vi "ge_RemoveArrayDup(String).vi"(4 "Input Array":string[](array[string])) -> (1 "Output Array":string[](array[string]))   [LabVIEW 2018]
doc: "This polymorphic VI removes all duplicate elements in <B>Input Array</B> and outputs the result as <B>Output Array</B>. It also outputs the <B>indices of removed elements<B>."
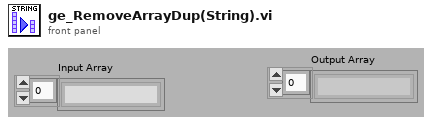
[diagram p1: front panel]
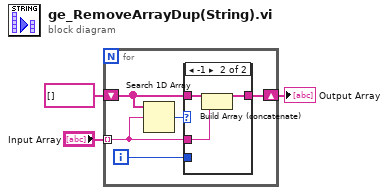
[diagram p0: block diagram]
diagram:
  n1 = for {
    tunnel: "Input Array" -> [w7] mode=indexing
    shift-right: [w6] -> w1
    shift-left: string[] [] -> [w5]
    i -> [w4]
    n2 = Search 1D Array(1D array=w5, element=w7) -> (index of element=w8:i32)  [unwired: 1 in]
    n3 = case shown="-1" w8 {
      tunnel: w7 -> [_ w12]
      tunnel: [w9 w10] -> w6
      tunnel: w5 -> [w9 w11]
      tunnel: w4 -> [_ _]
      frame Default {
      }
      frame -1 {
        n4 = Build Array (concatenate)(w11, w12) -> (w10:string[])
      }
    }
  }
  "Output Array" <- w1
